vi "Parse Multi Channel Data and Log.vi"(8 "error in":errorcluster, 10 "Variant":variant, 11 "Report in":refnum<class "Report.lvclass">) -> (0 "error out":errorcluster, 3 "Report out":refnum<class "Report.lvclass">)   [LabVIEW 2023, in "Report.lvlib" / "Report.lvclass"]
doc: "This should be a variant containing a string named Group and an array of waveforms. This routine converts the variant to the appropriate data and calls the write multi channel data override routine."
uses:
  Report.lvclass
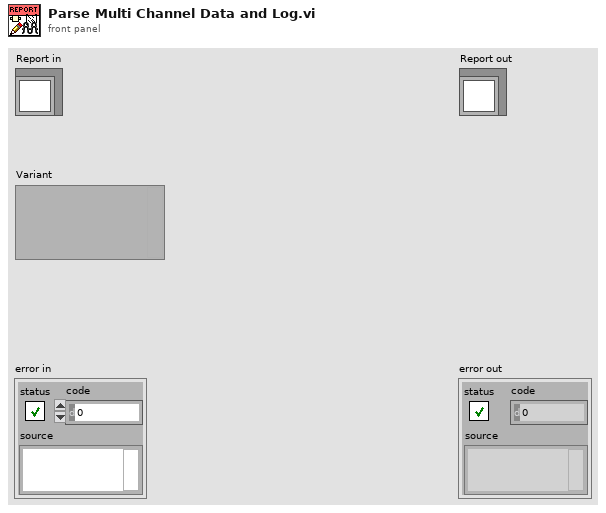
[diagram p1: front panel]
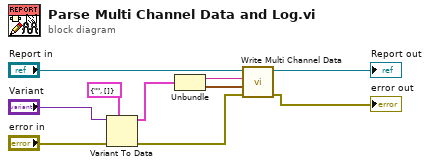
[diagram p0: block diagram]
diagram:
  n1 = Variant To Data(error in="error in", type=cluster{"Group":string, "Data":waveform(dbl)[]} {"Group"="", "Data"=[]} ("NChanMsg"), Variant="Variant") -> (data=w5:cluster{"Group":string, "Data":waveform(dbl)[]}, error out=w2:errorcluster)
  n2 = Unbundle(w5) -> ("Group"=w4:string, "Data"=w3:waveform(dbl)[])
  n3 = call-dynamic "Write Multi Channel Data.vi"("error in"=w2, "Data"=w3, "Group"=w4, "Report in"="Report in") -> ("error out"=→"error out":errorcluster, "Report out"=→"Report out":refnum<class "Report.lvclass">)  [unwired: 6 in]
